vi "STAGE+mono+counter_edit22.vi"() -> ()   [LabVIEW 2017]
panel:
  out "Timeout":bool
  out "PROGRESS":u8(slide) max=10 step=10 scale=0.0..1.0
  in  "?":enum32{"Scan Data", "Scans", "RT Data"}(tab)
  out "Spectrum":cluster{dbl[], dbl[]}(graph)
  out "Decay":cluster{dbl[], dbl[]}[](graph)
  in  "Collect Data!":bool
  out "Waveform Graph":waveform(dbl)[](graph)
  out "?":i32(knob) scale=0.0..1000000.0
  out "Photon Counts":dbl
  in  "Wavelength":dbl
  in  "Show Real Time Data":bool
  in  "?":enum32{"DELAY", "COUNTER", "MONO", "PLOT"}(tab)
  in  "Data File Path":path
  out "Final time [ps]":dbl
  out "Current time [ps]":dbl
  out "Initial time [ps]":dbl
  in  "Set this as t0":bool
  in  "Axis":i32=1
  in  "Motor ON":bool
  in  "Motor OFF":bool
  out "Current Position [mm]":dbl
  out "Final Position [mm]":dbl
  in  "Data Points":i32=100
  out "Current Point":i32
  in  "Step Size [um]":i32=10
  in  "Target [mm]":dbl format="%.3f"
  in  "Move":bool
  out "Initial position [mm]":dbl
  in  "GPIB address":string="23"
  in  "Count Mode":u16(ring) items=["A,B for Preset T", "A-B for Preset T", "A+B for Preset T", "A for Preset B"]
  in  "Trigger mode":u16(ring) items=["10 MHz"=0, "Input 2"=2, "Input T"=3]
  in  "Channel A Input":u16(ring)=1 items=["10 MHz", "Input 1"]
  in  "Channel B Input":u16(ring)=2 items=["Input 1"=1, "Input 2"=2]
  in  "Number of Measurements\n to take at one point/ Number of Periods":u16=1 min=1 max=2000 step=1
  in  "Time between measurements\n at one point (s)/Dwell Time":dbl=0.002 min=0.002 max=60.0 step=0.001
  in  "gate mode (CW:0)":i16(slide) scale=0.0..2.0 scale format="%.2f"
  out "Counts":i32
  in  "Integrating time \nin 10^-7 sec":dbl=10000000.0
  in  "Discriminator Level (mV)":dbl min=-300.0 max=300.0 step=0.2
  in  "Discriminator Slope":bool
  in  "Channel":i16 min=0 max=2 step=1
  out "Grating #":dbl
  out "Blaze angle":dbl
  out "Grooves/mm":dbl
  out "Mono port":T1(ring)
  out "Time delay":u32=450000 min=1
  in  "Step size":dbl=10.0 min=0.0
  in  "Scan to":i32=4000
  in  "Scan from":i32=2600
  out "Current wavelength":dbl
  in  "?":bool
  in  "Array":dbl[](array[numeric])
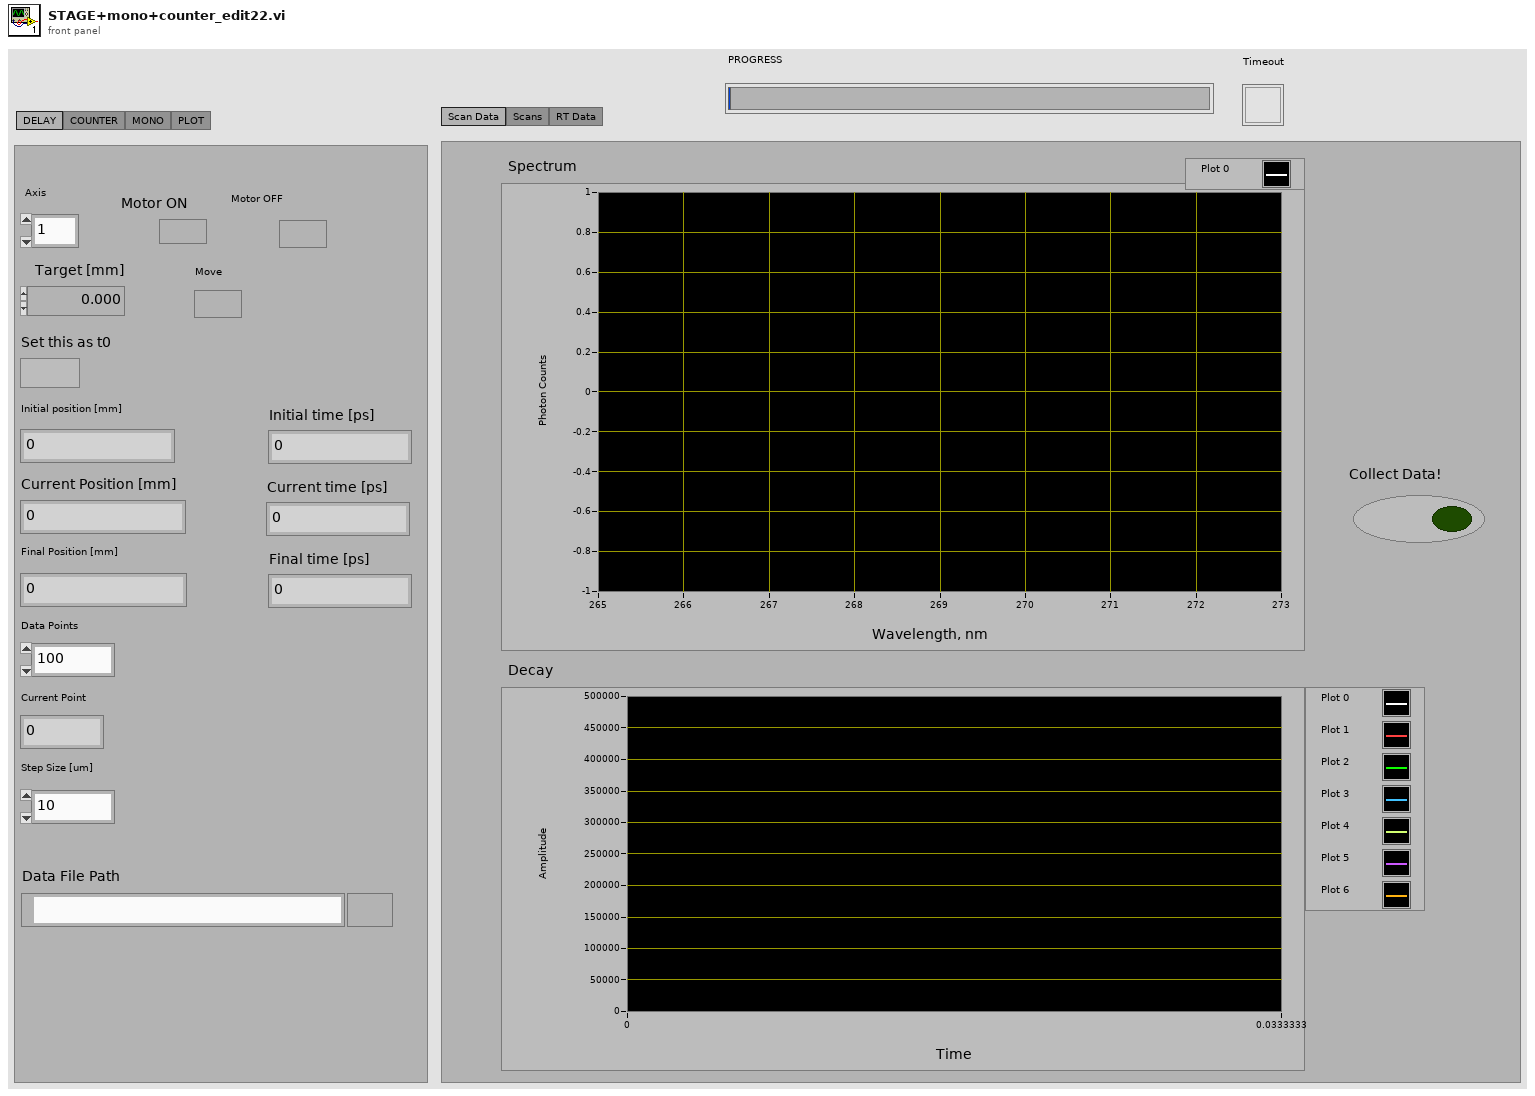
[diagram p1: front panel]
types:
  T1 = enum8{"COM 1", "COM 2", "COM 3", "COM 4", "COM 5", "COM 6", "COM 7", "COM 8", "COM 9"}
  T2 = cluster{"input XON/XOFF":bool, "input HW Handshake":bool, "input alt HW HShk":bool, "output XON/XOFF":bool, "output HW Handshake":bool, "output alt HW HShk":bool, "XOFF byte":u8, "XON byte":u8, "parity error byte":u16}
  T3 = enum16{"no parity", "odd parity", "even parity", "mark parity", "space parity"}
  T4 = enum16{"open", "replace", "create", "open or create", "replace or create", "replace or create with confirmation"}
  T5 = typedef "NI_Matrix.lvlib/RealMatrix.ctl" = dbl[][]
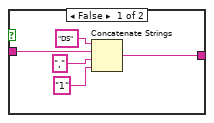
[diagram p3: hidden frame]
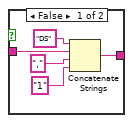
[diagram p5: hidden frame]
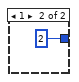
[diagram p9: hidden frame]
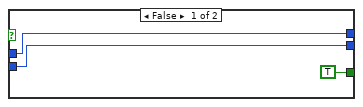
[diagram p10: hidden frame]
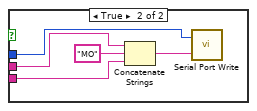
[diagram p11: hidden frame]
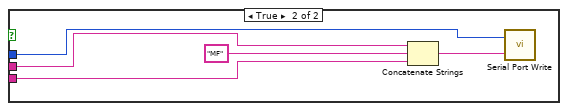
[diagram p12: hidden frame]
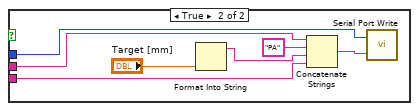
[diagram p13: hidden frame]
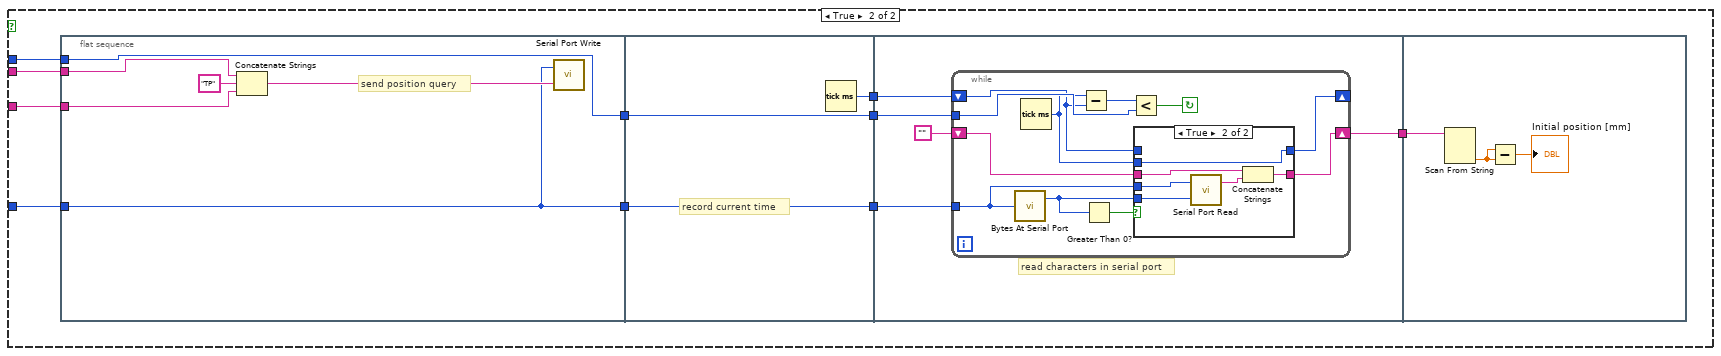
[diagram p14: hidden frame]
diagram:
  (unwired) FALSE
  w28 = u32 19200  # baud rate
  w27 = u16 8  # data bits
  w26 = enum16{"1 bit", "1.5 bits", "2 bits"}."1 bit"  # stop bits
  w30 = T3."no parity"  # parity
  w6 = 4  # 0=COM1 so n=COM(n+1)
  w29 = u16 1024  # buffer size
  n1 = flat-sequence {
    tunnel: [w33] -> w21
    tunnel: [w32] -> w20
    frame #0 {
      n2 = call "CM Com Read ini.vi"() -> ("Mono port"=w32:T1, "time delay1"=w33:u32)  [unwired: 7 in]
    }
  }
  n3 = call "CM Serial Port Setup.vi"("COM port"=w20, "time delay"=w21) -> ("time delay1"=w16:u32, "DK port Out"=w17:T1, "error code"=w19:i32)  [unwired: 7 in]
  n4 = Equal To 0?(x=w19) -> (x = 0?=w18:bool)
  n5 = case shown="True" w18 {
    tunnel: w17 -> [w36 w39]
    tunnel: w16 -> [w35 w38]
    tunnel: [w36 w39] -> w3
    tunnel: [w35 w38] -> w2
    tunnel: [TRUE FALSE] -> w1
    frame False {
    }
    frame True {
      n6 = call "CM Com Write ini.vi"("time delay1"=w39, "Mono port"=w38) -> ()  [unwired: 7 in]
      n7 = local write "Mono port"(w39) -> ()
      n8 = local write "Time delay"(w38) -> ()
    }
  }
  n9 = call <vilib>:"Serial Port Init.vi"("flow control etc."=T2 {"input XON/XOFF"=FALSE, "input HW Handshake"=FALSE, "input alt HW HShk"=FALSE, "output XON/XOFF"=FALSE, "output HW Handshake"=FALSE, "output alt HW HShk"=FALSE, "XOFF byte"=13, "XON byte"=11, "parity error byte"=0}, "parity"=w30, "buffer size"=w29, "stop bits"=w26, "data bits"=w27, "baud rate"=w28, "port number"=w6) -> ("error code"=w25:i32)
  n10 = Concatenate Strings("\r", "\n") -> (w22:string)
  n11 = while {
    tunnel: w2 -> [w42]
    tunnel: w3 -> [w41]
    stop <- TRUE continue-if-true
    n12 = case shown="True" "?" {
      tunnel: w42 -> [_ w45]
      tunnel: w41 -> [_ w44]
      frame False {
      }
      frame True {
        n13 = Two Button Dialog(message="Do you want to change grating?", 1:"No" ("F button name (\"Cancel\")"), 2:"Yes" ("T button name (\"OK\")")) -> (T button?=w46:bool)
        n14 = case shown="True" w46 {
          tunnel: w45 -> [_ w51]
          tunnel: w44 -> [_ w50]
          frame False {
          }
          frame True {
            n15 = Two Button Dialog(message="Disable voltage from PMT", 1:"Do not swich grating" ("F button name (\"Cancel\")"), 2:"Done" ("T button name (\"OK\")")) -> (T button?=w52:bool)
            n16 = case shown="True" w52 {
              tunnel: w51 -> [_ w64]
              tunnel: w50 -> [_ w63]
              frame False {
              }
              frame True {
                n17 = flat-sequence {
                  tunnel: w64 -> [w68]
                  tunnel: [w68] -> w58
                  tunnel: w63 -> [w67]
                  tunnel: [w67] -> w57
                  tunnel: [w65] -> w56
                  tunnel: w58 -> [w73]
                  tunnel: [w73] -> w61
                  tunnel: w57 -> [w74]
                  tunnel: [w74] -> w60
                  tunnel: w56 -> [w72]
                  tunnel: [w72] -> w59
                  tunnel: w61 -> [w78]
                  tunnel: w60 -> [w79]
                  tunnel: [w77] -> w62
                  tunnel: w59 -> [w77]
                  frame #0 {
                    n18 = local read "Grating #"() -> (w66:dbl)
                    n19 = case shown="2, Default" w66 {
                      tunnel: [1 2] -> w65
                      frame 2, Default {
                      }
                      frame 1 {
                      }
                    }
                    n20 = call "Select11x2.vi"("time delay"=w68, "NEW GRT?"=w65, "port number"=w67) -> ()  [unwired: 3 out]
                  }
                  frame #1 {
                    n21 = call "Query11x.vi"("port number"=w74, "QUERY"=u16 2, "time delay"=w73) -> ("STATUS MESSAGE"=w71:u16)  [unwired: 3 out]
                    n22 = local write "Grooves/mm"(w71) -> ()
                  }
                  frame #2 {
                    n23 = Divide(x=w78, y=i16 100 ("device (1)")) -> (x/y=w80:dbl)
                    n24 = call "Query11x.vi"("port number"=w79, "QUERY"=u16 3, "time delay"=w80) -> ("STATUS MESSAGE"=w76:u16)  [unwired: 3 out]
                    n25 = local write "Blaze angle"(w76) -> ()
                  }
                }
                n26 = local write "Grating #"(w62) -> ()
              }
            }
          }
        }
      }
    }
  }
  n27 = while {
    tunnel: w6 -> [w97]
    tunnel: w22 -> [w98]
    tunnel: w25 -> [_]
    tunnel: "Axis" -> [w95]
    stop <- TRUE continue-if-true
    w96 = u32 200  # timeout
    n28 = Format Into String(w95) -> (resulting string=w99:string)  [unwired: 3 in, 1 out]
    n29 = flat-sequence {
      tunnel: w99 -> [w104]
      tunnel: w98 -> [w103]
      tunnel: w97 -> [w105]
      tunnel: w96 -> [w102]
      tunnel: [w104] -> w94
      tunnel: [w103] -> w93
      tunnel: [w105] -> w92
      tunnel: [w102] -> w91
      tunnel: w94 -> [w115]
      tunnel: w93 -> [w114]
      tunnel: w92 -> [w116]
      tunnel: w91 -> [w112]
      tunnel: [w115] -> w90
      tunnel: [w114] -> w89
      tunnel: [w116] -> w88
      tunnel: [w112] -> w87
      tunnel: w90 -> [w125]
      tunnel: w89 -> [w124]
      tunnel: w88 -> [w126]
      tunnel: w87 -> [w122]
      tunnel: [w125] -> w86
      tunnel: [w124] -> w85
      tunnel: [w126] -> w84
      tunnel: [w122] -> w83
      tunnel: w86 -> [w138]
      tunnel: w85 -> [w135]
      tunnel: w84 -> [w137]
      tunnel: w83 -> [w136]
      frame #0 {
        n30 = case shown="False" "Motor ON" {
          tunnel: w105 -> [_ w111]
          tunnel: w104 -> [_ w108]
          tunnel: w103 -> [_ w107]
          frame False {
          }
          frame True {
            n31 = Concatenate Strings(w108, "MO" ("Substring"), w107) -> (w109:string)
            n32 = call <vilib>:"Serial Port Write.vi"("string to write"=w109, "port number"=w111) -> ()  [unwired: 1 out]
          }
        }
      }
      frame #1 {
        n33 = case shown="False" "Motor OFF" {
          tunnel: w116 -> [_ w121]
          tunnel: w115 -> [_ w118]
          tunnel: w114 -> [_ w117]
          frame False {
          }
          frame True {
            n34 = Concatenate Strings(w118, "MF" ("Substring"), w117) -> (w119:string)
            n35 = call <vilib>:"Serial Port Write.vi"("string to write"=w119, "port number"=w121) -> ()  [unwired: 1 out]
          }
        }
      }
      frame #2 {
        n36 = case shown="False" "Move" {
          tunnel: w126 -> [_ w133]
          tunnel: w125 -> [_ w130]
          tunnel: w124 -> [_ w129]
          frame False {
          }
          frame True {
            n37 = Format Into String("Target [mm]") -> (resulting string=w127:string)  [unwired: 3 in, 1 out]
            n38 = Concatenate Strings(w130, "PA" ("Substring"), w127, w129) -> (w131:string)
            n39 = call <vilib>:"Serial Port Write.vi"("string to write"=w131, "port number"=w133) -> ()  [unwired: 1 out]
          }
        }
      }
      frame #3 {
        n40 = case shown="False" "Set this as t0" {
          tunnel: w138 -> [_ w148]
          tunnel: w137 -> [_ w147]
          tunnel: w136 -> [_ w146]
          tunnel: w135 -> [_ w145]
          frame False {
          }
          frame True {
            n41 = flat-sequence {
              tunnel: w148 -> [w152]
              tunnel: w147 -> [w151]
              tunnel: [w151] -> w144
              tunnel: w146 -> [w149]
              tunnel: [w149] -> w143
              tunnel: w145 -> [w150]
              tunnel: w144 -> [w156]
              tunnel: [w156] -> w142
              tunnel: w143 -> [w155]
              tunnel: [w155] -> w141
              tunnel: [w157] -> w140
              tunnel: w142 -> [w162]
              tunnel: w141 -> [w160]
              tunnel: w140 -> [w159]
              tunnel: [w158] -> w139
              tunnel: w139 -> [w184]
              frame #0 {
                # "send position query"
                n42 = Concatenate Strings(w152, "TP" ("Substring"), w150) -> (w153:string)
                n43 = call <vilib>:"Serial Port Write.vi"("string to write"=w153, "port number"=w151) -> ()  [unwired: 1 out]
              }
              frame #1 {
                # "record current time"
                n44 = Tick Count (ms)() -> (millisecond timer value=w157:u32)
              }
              frame #2 {
                # "read characters in serial port"
                n45 = while {
                  shift-left: w159 -> [w163]
                  shift-right: [w164] -> _
                  tunnel: w160 -> [w167]
                  shift-left: "" -> [w170]
                  shift-right: [w169] -> w158
                  tunnel: w162 -> [w171]
                  stop <- w166 continue-if-true
                  n46 = call <vilib>:"Bytes At Serial Port.vi"("port number"=w171) -> ("byte count"=w172:u32)  [unwired: 1 out]
                  n47 = Tick Count (ms)() -> (millisecond timer value=w165:u32)
                  n48 = Subtract(x=w165, y=w163) -> (x-y=w168:u32)
                  n49 = Greater Than 0?(x=w172) -> (x > 0?=w173:bool)
                  n50 = Less?(x=w168, y=w167) -> (x < y?=w166:bool)
                  n51 = case shown="True" w173 {
                    tunnel: w172 -> [_ w181]
                    tunnel: w171 -> [_ w180]
                    tunnel: w170 -> [w175 w178]
                    tunnel: [w175 w177] -> w169
                    tunnel: [w174 w176] -> w164
                    tunnel: w165 -> [_ w176]
                    tunnel: w163 -> [w174 _]
                    frame False {
                    }
                    frame True {
                      n52 = call <vilib>:"Serial Port Read.vi"("requested byte count"=w181, "port number"=w180) -> ("string read"=w179:string)  [unwired: 1 out]
                      n53 = Concatenate Strings(w178, w179) -> (w177:string)
                    }
                  }
                }
              }
              frame #3 {
                n54 = Scan From String(input string=w184) -> (output 1=w182:dbl)  [unwired: 4 in, 3 out]
                n55 = Subtract(x=w182, y=w182) -> (x-y=→"Initial position [mm]":dbl)
              }
            }
          }
        }
      }
    }
    n56 = Wait Until Next ms Multiple(millisecond multiple=u32 50) -> ()  [unwired: 1 out]
  }
  n57 = while {
    tunnel: "GPIB address" -> [w188]
    tunnel: w3 -> [w187]
    tunnel: w2 -> [w186]
    tunnel: w1 -> [w185]
    stop <- TRUE continue-if-true
    n58 = case shown="True" "Show Real Time Data" {
      tunnel: w188 -> [_ w195]
      tunnel: w187 -> [_ w194]
      tunnel: w186 -> [_ w193]
      tunnel: w185 -> [_ w192]
      frame False {
      }
      frame True {
        n59 = flat-sequence {
          tunnel: w195 -> [w224]
          tunnel: "Wavelength" -> [w225]
          tunnel: [w225] -> w206
          tunnel: [w214] -> w205
          tunnel: [w213] -> w204
          tunnel: [w224] -> w203
          tunnel: w193 -> [w217]
          tunnel: w194 -> [w216]
          tunnel: w192 -> [w215]
          tunnel: [w264] -> w202
          tunnel: [w263] -> w201
          tunnel: [w261] -> w200
          tunnel: w206 -> [w259]
          tunnel: w205 -> [w264]
          tunnel: w204 -> [w263]
          tunnel: w203 -> [w261]
          tunnel: w202 -> [w271]
          tunnel: w201 -> [w270]
          tunnel: w200 -> [w265]
          tunnel: [w265] -> w199
          tunnel: w199 -> [w276]
          tunnel: [w276] -> w198
          tunnel: w198 -> [w326]
          tunnel: [w326] -> w197
          tunnel: w197 -> [w327]
          tunnel: [w327] -> w196
          tunnel: w196 -> [w337]
          frame #0 {
            n60 = flat-sequence {
              tunnel: w217 -> [w231]
              tunnel: [w231] -> w223
              tunnel: w216 -> [w233]
              tunnel: [w233] -> w222
              tunnel: w215 -> [w229]
              tunnel: [w229] -> w221
              tunnel: w223 -> [w237]
              tunnel: [w237] -> w212
              tunnel: w222 -> [w238]
              tunnel: [w238] -> w210
              tunnel: w221 -> [w235]
              tunnel: [w235] -> w208
              tunnel: w212 -> [w242]
              tunnel: [w242] -> w211
              tunnel: w210 -> [w241]
              tunnel: [w241] -> w209
              tunnel: w208 -> [w240]
              tunnel: [w240] -> w207
              tunnel: w211 -> [w249]
              tunnel: [w249] -> w220
              tunnel: w209 -> [w246]
              tunnel: [w246] -> w219
              tunnel: w207 -> [w244]
              tunnel: [w244] -> w218
              tunnel: w220 -> [w252]
              tunnel: w219 -> [w253]
              tunnel: w218 -> [_]
              tunnel: [w253] -> w214
              tunnel: [w252] -> w213
              frame #0 {
                n61 = call "Query11x.vi"("port number"=w233, "QUERY"=u16 0, "time delay"=w231) -> ("timeout"=w230:bool, "STATUS MESSAGE"=w228:u16)  [unwired: 2 out]
                n62 = local write "Timeout"(w230) -> ()
                n63 = Divide(x=w228, y=10 ("Numeric")) -> (x/y=w226:dbl)
                n64 = local write "Current wavelength"(w226) -> ()
              }
              frame #1 {
                n65 = call "Query11x.vi"("port number"=w238, "QUERY"=u16 2, "time delay"=w237) -> ("timeout"=w236:bool, "STATUS MESSAGE"=w234:u16)  [unwired: 2 out]
                n66 = local write "Timeout"(w236) -> ()
                n67 = local write "Grooves/mm"(w234) -> ()
              }
              frame #2 {
              }
              frame #3 {
                n68 = Divide(x=w249, y=i16 100 ("device (1)")) -> (x/y=w247:dbl)
                n69 = call "Query11x.vi"("port number"=w246, "QUERY"=u16 3, "time delay"=w247) -> ("timeout"=w245:bool, "STATUS MESSAGE"=w243:u16)  [unwired: 2 out]
                n70 = local write "Timeout"(w245) -> ()
                n71 = local write "Blaze angle"(w243) -> ()
              }
              frame #4 {
                n72 = Divide(x=w252, y=i16 100 ("device (1)")) -> (x/y=w255:dbl)
                n73 = call "Query11x.vi"("port number"=w253, "QUERY"=u16 4, "time delay"=w255) -> ("timeout"=w254:bool, "STATUS MESSAGE"=w251:u16)  [unwired: 2 out]
                n74 = local write "Timeout"(w254) -> ()
                n75 = local write "Grating #"(w251) -> ()
              }
            }
          }
          frame #1 {
            n76 = Multiply(x=w259, y=1) -> (x*y=w258:dbl)
            n77 = call "Goto11x.vi"("time delay"=w263, "WAVELENGTH"=w258, "port number"=w264) -> ("timeout"=w262:bool)  [unwired: 2 out]
            n78 = local write "Timeout"(w262) -> ()
          }
          frame #2 {
            # "set counter time in 10^-7 seconds in CW"
            n79 = call "Query11x.vi"("port number"=w271, "QUERY"=0, "time delay"=w270) -> ("timeout"=w269:bool, "STATUS MESSAGE"=w268:u16)  [unwired: 2 out]
            n80 = local write "Timeout"(w269) -> ()
            n81 = Divide(x=w268, y=1) -> (x/y=w267:dbl)
            n82 = local write "Current wavelength"(w267) -> ()
          }
          frame #3 {
            # "Configures discriminator."
            n83 = flat-sequence {
              tunnel: w276 -> [w283]
              tunnel: [w283] -> w282
              tunnel: [w290] -> w281
              tunnel: [w288] -> w280
              tunnel: w275 -> [w289]
              tunnel: w282 -> [w288]
              tunnel: w277 -> [w287]
              tunnel: w281 -> [w309]
              tunnel: [w310] -> w279
              tunnel: w280 -> [w308]
              tunnel: [w308] -> w278
              tunnel: w277 -> [w306]
              tunnel: w279 -> [w322]
              tunnel: w278 -> [w321]
              tunnel: w273 -> [w316]
              tunnel: w277 -> [w315]
              frame #0 {
                # "Flush I/O buffers."
                n84 = for {
                  N: 5 -> [_]
                  tunnel: w283 -> [w285]
                  n85 = GPIB Write(0:w285, 1:"\r") -> ()  [unwired: 3 in, 2 out]
                }
              }
              frame #1 {
                # "Set discriminator slope."
                n86 = case shown="True" w289 {
                  tunnel: [w296 w301] -> w291
                  tunnel: w287 -> [w295 w300]
                  frame False {
                    n87 = Concatenate Strings("DS", w295, ",", "1") -> (w296:string)
                  }
                  frame True {
                    n88 = Concatenate Strings("DS", w300, ",", "0") -> (w301:string)
                  }
                }
                n89 = GPIB Write(0:w288, 1:w291, 2:5) -> (6:w290:errorcluster)  [unwired: 2 in, 1 out]
              }
              frame #2 {
                # "Set discriminator mode to fixed."
                n90 = Concatenate Strings("DM", w306, ",", "0") -> (w305:string)
                n91 = GPIB Write(0:w308, 1:w305, 2:5, 3:w309) -> (6:w310:errorcluster)  [unwired: 1 in, 1 out]
              }
              frame #3 {
                # "Set discriminator level.\nMust be between +300 and -300 mV."
                n92 = Divide(x=w316, y=1000.0) -> (x/y=w324:dbl)
                n93 = Number To Fractional String(number=w324, precision (6)=i16 4) -> (F-format string=w313:string)  [unwired: 2 in]
                n94 = Concatenate Strings("DL", w315, ",", w313) -> (w320:string)
                n95 = GPIB Write(0:w321, 1:w320, 2:5, 3:w322) -> (6:w317:errorcluster)  [unwired: 1 in, 1 out]
                n96 = call <vilib>:"General Error Handler.vi"("type of dialog (OK msg:1)"=1, "error in (no error)"=w317) -> ()  [unwired: 9 in, 5 out]
              }
            }
            n97 = local read "Discriminator Slope"() -> (w275:bool)
            n98 = local read "Channel"() -> (w274:i16)
            n99 = Number To Decimal String(number=w274) -> (decimal integer string=w277:string)  [unwired: 1 in]
            n100 = local read "Discriminator Level (mV)"() -> (w273:dbl)
          }
          frame #4 {
            n101 = call "Start.vi"("GPIB Address"=w326) -> ()  [unwired: 9 in]
          }
          frame #5 {
            # "Wait for Scan to Finish"
            n102 = for {
              N: 1 -> [_]
              tunnel: w327 -> [w329]
              n103 = while {
                tunnel: w329 -> [w330]
                stop <- w332 stop-if-true
                n104 = call "ScanDone.vi"("Wait (ms)"=1000, "GPIB Address"=w330) -> ("Scan Finished?"=w332:bool)
              }
            }
          }
          frame #6 {
            n105 = call "Read Data.vi"("Channel Number"=0, "GPIB Address"=w337, "Number of Datapoints"=1) -> ("Data"=w338:i32[])
            n106 = property class="Knob (strict)"("Scale.Increment"=1000, "Scale.Maximum"=1000000, "Scale.Minimum"=0) -> ()  [unwired: 2 in, 2 out]
            n107 = Index Array(array=w338, index=0) -> (element=→"Photon Counts" →"?":i32)
          }
        }
      }
    }
  }
  n108 = while {
    tunnel: "Axis" -> [w350]
    tunnel: w6 -> [w349]
    tunnel: "GPIB address" -> [w348]
    tunnel: "Integrating time \nin 10^-7 sec" -> [w347]
    tunnel: w2 -> [w346]
    tunnel: w3 -> [w345]
    tunnel: w1 -> [w344]
    stop <- TRUE continue-if-true
    n109 = case shown="True" "Collect Data!" {
      selector: "Collect Data!" -> [_ w351]
      tunnel: w350 -> [_ w359]
      tunnel: w349 -> [_ w358]
      tunnel: w348 -> [_ w357]
      tunnel: w348 -> [_ w355]
      tunnel: w347 -> [_ w354]
      tunnel: w346 -> [_ w353]
      tunnel: w345 -> [_ w356]
      tunnel: w344 -> [_ w352]
      frame False {
      }
      frame True {
        n110 = flat-sequence {
          tunnel: w359 -> [w379]
          tunnel: w358 -> [w377]
          tunnel: w357 -> [w376]
          tunnel: w356 -> [w375]
          tunnel: w355 -> [w374]
          tunnel: w354 -> [w371]
          tunnel: w353 -> [w364]
          tunnel: w352 -> [w363]
          tunnel: w351 -> [_]
          frame #0 {
            w384 = 1000000000000.0
            w389 = 1000
            w390 = 300000000
            w396 = 1
            n111 = Multiply(x="Step Size [um]", y="Data Points") -> (x*y=w393:i32)
            n112 = Divide(x="Step Size [um]", y=1000.0) -> (x/y=w402:dbl)
            n113 = local read "Initial position [mm]"() -> (w381:dbl)
            n114 = Increment(x="Data Points") -> (x+1=w411:i32)
            n115 = Multiply(x="Scan to", y=w396) -> (x*y=w370:i32)
            n116 = Multiply(x="Scan from", y=w396) -> (x*y=w369:i32)
            n117 = Divide(x=w393, y=1000) -> (x/y=w392:dbl)
            n118 = To Time Stamp(1:w369) -> (0:w399:timestamp)
            n119 = Multiply(x=w370, y=1) -> (x*y=w408:i32)
            n120 = Multiply(x=1, y=w369) -> (x*y=w373:i32)
            n121 = Divide(x=w402, y=1000.0) -> (x/y=w403:dbl)
            n122 = for {
              N: w411 -> [_]
              tunnel: w402 -> [w809]
              tunnel: w381 -> [w807]
              tunnel: [w800] -> w410 mode=indexing
              i -> [w808]
              # "distances"
              n123 = Multiply(x=w809, y=w808) -> (x*y=w806:dbl)
              n124 = Add(x=w807, y=w806) -> (x+y=w805:dbl)
              n125 = Divide(x=w805, y=1000) -> (x/y=w799:dbl)
              n126 = Divide(x=w799, y=300000000) -> (x/y=w802:dbl)
              n127 = Multiply(x=w802, y=1000000000000.0) -> (x*y=w800:dbl)
            }
            n128 = Subtract(x=w408, y=w373) -> (x-y=w414:i32)
            n129 = Divide(x=w381, y=w389) -> (x/y=w387:dbl)
            n130 = Add(x=w381, y=w392) -> (x+y=w383:dbl)
            "Final Position [mm]" <- w383
            n131 = property on="Waveform Graph" class="WFGraph (strict)"("XScale.Increment"="Step size", "XScale.Maximum"=w370, "XScale.Minimum"=w369) -> ()  [unwired: 2 in, 2 out]
            n132 = Divide(x=w383, y=w389) -> (x/y=w388:dbl)
            n133 = Divide(x=w414, y="Step size") -> (x/y=w413:dbl)
            n134 = Divide(x=w387, y=w390) -> (x/y=w386:dbl)
            n135 = Divide(x=w403, y=300000000) -> (x/y=w405:dbl)
            n136 = Bundle By Name("Y"=dbl[] [], "t0"=w399, "dt"="Step size") -> (w398:waveform(dbl))  [unwired: 1 in]
            n137 = Divide(x=w388, y=w390) -> (x/y=w385:dbl)
            n138 = Multiply(x=w405, y=1000000000000.0) -> (x*y=w367:dbl)
            n139 = Multiply(x=w386, y=w384) -> (x*y=w366:dbl)
            "Initial time [ps]" <- w366
            n140 = Build Array(w398) -> (w362:waveform(dbl)[])
            n141 = Round Toward -Infinity(1:w413) -> (0:w372:dbl)
            n142 = Concatenate Strings("\r", "\n") -> (w378:string)
            n143 = Increment(x=w372) -> (x+1=w401:dbl)
            n144 = Multiply(x=w385, y=w384) -> (x*y=w397:dbl)
            "Final time [ps]" <- w397
            n145 = for {
              N: w401 -> [_]
              tunnel: "Step size" -> [w814]
              tunnel: w373 -> [w812]
              tunnel: [w810] -> _ mode=indexing
              i -> [w813]
              # "wavelengths"
              n146 = Multiply(x=w814, y=w813) -> (x*y=w811:dbl)
              n147 = Add(x=w812, y=w811) -> (x+y=w810:dbl)
            }
            n148 = for {
              N: "Data Points" -> [w438]
              tunnel: w381 -> [w479]
              tunnel: "Step Size [um]" -> [w475]
              tunnel: w379 -> [w472]
              tunnel: w378 -> [w469]
              tunnel: w377 -> [w470]
              tunnel: w376 -> [w468]
              tunnel: w375 -> [w466]
              tunnel: w374 -> [w467]
              tunnel: w373 -> [w429]
              tunnel: "Step size" -> [w461]
              tunnel: w372 -> [w460]
              tunnel: w371 -> [w459]
              tunnel: w370 -> [w424]
              tunnel: w369 -> [w423]
              tunnel: "Step size" -> [w425]
              tunnel: w367 -> [w440]
              tunnel: w366 -> [w457]
              shift-right: [w439] -> _
              shift-left: dbl[] [] -> [w435]
              tunnel: w364 -> [w452]
              tunnel: w375 -> [w451]
              tunnel: w363 -> [w450]
              shift-right: [w445] -> _
              shift-left: w362 -> [w446]
              shift-right: [w433] -> _
              shift-left: dbl[][] [] -> [w432]
              shift-right: [w421] -> _
              shift-left: dbl[][] [] -> [w419]
              i -> [w427]
              w449 = dbl[] []
              n149 = property on="PROGRESS" class="Slide (strict)"("Scale.Increment"=1, "Scale.Maximum"=w438, "Scale.Minimum"=0) -> ()  [unwired: 2 in, 2 out]
              n150 = stacked-sequence {
                tunnel: w466 -> [w782]
                tunnel: w467 -> [_]
                frame #0 {
                  n151 = call <vilib>:"Close Serial Driver.vi"("port number"=w782) -> ()  [unwired: 1 out]
                  n152 = GPIB Misc(0:"loc 23" ("command string")) -> ()  [unwired: 1 in, 3 out]
                }
              }
              n153 = property on="Waveform Graph" class="WFGraph (strict)"("XScale.Increment"=w425, "XScale.Maximum"=w424, "XScale.Minimum"=w423) -> ()  [unwired: 2 in, 2 out]
              n154 = Multiply(x=w440, y=w427) -> (x*y=w458:dbl)
              n155 = Number To Decimal String(number=w459) -> (decimal integer string=w464:string)  [unwired: 1 in]
              n156 = Add(x=1, y=w427) -> (x+y=→"PROGRESS":i32)
              n157 = Divide(x=w475, y=1000) -> (x/y=w474:dbl)
              n158 = Add(x=w457, y=w458) -> (x+y=w436:dbl)
              n159 = Concatenate Strings("CP 2,", w464) -> (w462:string)
              n160 = Multiply(x=w474, y=w427) -> (x*y=w478:dbl)
              n161 = Build Array (concatenate)(w435, w436) -> (w437:dbl[])
              n162 = Add(x=w479, y=w478) -> (x+y=w477:dbl)
              n163 = Format Into String(w472) -> (resulting string=w471:string)  [unwired: 3 in, 1 out]
              n164 = GPIB Write(0:w468, 1:w462, 2:i16 5 ("mode (0)")) -> ()  [unwired: 2 in, 2 out]
              n165 = flat-sequence {
                tunnel: w477 -> [w785]
                tunnel: [w785] -> w473
                tunnel: w469 -> [w787]
                tunnel: w471 -> [w786]
                tunnel: w470 -> [w783]
                tunnel: w473 -> [w796]
                tunnel: [w791] -> w422
                frame #0 {
                  n166 = Format Into String(w785) -> (resulting string=w784:string)  [unwired: 3 in, 1 out]
                  n167 = Wait (ms)(milliseconds to wait=u32 100) -> ()  [unwired: 1 out]
                  n168 = Concatenate Strings(w786, "PA" ("Substring"), w784, w787) -> (w789:string)
                  n169 = call <vilib>:"Serial Port Write.vi"("string to write"=w789, "port number"=w783) -> ()  [unwired: 1 out]
                }
                frame #1 {
                  n170 = Divide(x=w796, y=1000) -> (x/y=w794:dbl)
                  n171 = Wait (ms)(milliseconds to wait=u32 1000) -> ()  [unwired: 1 out]
                  n172 = Divide(x=w794, y=300000000) -> (x/y=w793:dbl)
                  n173 = Multiply(x=w793, y=1000000000000.0) -> (x*y=w791:dbl)
                  "Current time [ps]" <- w791
                  "Current Position [mm]" <- w796
                }
              }
              n174 = Add(x=w427, y=1) -> (x+y=w426:i32)
              n175 = flat-sequence {
                tunnel: w468 -> [w505]
                tunnel: w429 -> [w504]
                tunnel: w461 -> [w503]
                tunnel: w460 -> [w502]
                tunnel: w424 -> [w501]
                tunnel: w423 -> [w500]
                tunnel: w449 -> [w499]
                tunnel: w449 -> [w498]
                tunnel: w425 -> [w497]
                tunnel: w452 -> [w496]
                tunnel: w451 -> [w495]
                tunnel: w450 -> [w494]
                tunnel: [w492] -> w448
                tunnel: [w493] -> _
                tunnel: [w492] -> w447
                tunnel: w426 -> [w491]
                tunnel: w422 -> [w490]
                tunnel: [w489] -> w420
                tunnel: w419 -> [w488]
                tunnel: w448 -> [w760]
                tunnel: [w763] -> w434
                tunnel: [w762] -> w431
                tunnel: [w761] -> w421
                tunnel: w420 -> [w761]
                frame #0 {
                  # "step size"
                  n176 = while {
                    tunnel: w505 -> [w545]
                    tunnel: w504 -> [w568]
                    tunnel: w503 -> [w538]
                    tunnel: w502 -> [w567]
                    tunnel: w501 -> [w541]
                    tunnel: w500 -> [w540]
                    tunnel: w497 -> [w542]
                    shift-right: [w564] -> w492
                    shift-left: w498 -> [w563]
                    shift-right: [w559] -> w493
                    shift-left: w499 -> [w566]
                    tunnel: w496 -> [w549]
                    tunnel: w495 -> [w548]
                    tunnel: w494 -> [w547]
                    tunnel: w491 -> [w526]
                    tunnel: w490 -> [w514]
                    shift-right: [w507] -> w489
                    shift-left: w488 -> [w506]
                    i -> [w534]
                    stop <- w536 stop-if-true
                    n177 = property on="Spectrum" class="XYGraph (strict)"("XScale.Increment"=w542, "XScale.Maximum"=w541, "XScale.Minimum"=w540) -> ()  [unwired: 2 in, 2 out]
                    n178 = Multiply(x=1, y=w538) -> (x*y=w537:dbl)
                    n179 = Greater Or Equal?(x=w534, y=w567) -> (x >= y?=w536:bool)
                    n180 = Multiply(x=w534, y=w537) -> (x*y=w569:dbl)
                    n181 = Add(x=w569, y=w568) -> (x+y=w546:dbl)
                    n182 = Add(x=w534, y=1) -> (x+y=w527:i32)
                    n183 = Build Array (concatenate)(w566, w546) -> (w565:dbl[])
                    n184 = flat-sequence {
                      tunnel: w545 -> [w590]
                      tunnel: w546 -> [w591]
                      tunnel: [w591] -> w553
                      tunnel: [w580] -> w552
                      tunnel: [w579] -> w551
                      tunnel: [w590] -> w550
                      tunnel: w549 -> [w583]
                      tunnel: w548 -> [w582]
                      tunnel: w547 -> [w581]
                      tunnel: [w572] -> w528
                      tunnel: w527 -> [w572]
                      tunnel: [w571] -> w515
                      tunnel: w514 -> [w571]
                      tunnel: w506 -> [w570]
                      tunnel: [w570] -> w513
                      tunnel: [w633] -> w558
                      tunnel: [w632] -> w557
                      tunnel: [w630] -> w556
                      tunnel: w553 -> [w626]
                      tunnel: w552 -> [w633]
                      tunnel: w551 -> [w632]
                      tunnel: w550 -> [w630]
                      tunnel: [w627] -> w529
                      tunnel: w528 -> [w627]
                      tunnel: [w626] -> w521
                      tunnel: [w625] -> w516
                      tunnel: w515 -> [w625]
                      tunnel: w513 -> [w624]
                      tunnel: [w624] -> w512
                      tunnel: w558 -> [w644]
                      tunnel: w557 -> [w643]
                      tunnel: w556 -> [w638]
                      tunnel: [w638] -> w544
                      tunnel: [w637] -> w530
                      tunnel: w529 -> [w637]
                      tunnel: [w636] -> w522
                      tunnel: w521 -> [w636]
                      tunnel: [w635] -> w517
                      tunnel: w516 -> [w635]
                      tunnel: w512 -> [w634]
                      tunnel: [w634] -> w511
                      tunnel: w544 -> [w650]
                      tunnel: [w650] -> w543
                      tunnel: [w649] -> w531
                      tunnel: w530 -> [w649]
                      tunnel: [w648] -> w523
                      tunnel: w522 -> [w648]
                      tunnel: [w647] -> w518
                      tunnel: w517 -> [w647]
                      tunnel: w511 -> [w646]
                      tunnel: [w646] -> w510
                      tunnel: w543 -> [w707]
                      tunnel: [w707] -> w555
                      tunnel: [w706] -> w532
                      tunnel: w531 -> [w706]
                      tunnel: [w705] -> w524
                      tunnel: w523 -> [w705]
                      tunnel: [w704] -> w519
                      tunnel: w518 -> [w704]
                      tunnel: w510 -> [w703]
                      tunnel: [w703] -> w509
                      tunnel: w555 -> [w712]
                      tunnel: [w712] -> w554
                      tunnel: [w711] -> w533
                      tunnel: w532 -> [w711]
                      tunnel: [w710] -> w525
                      tunnel: w524 -> [w710]
                      tunnel: [w709] -> w520
                      tunnel: w519 -> [w709]
                      tunnel: w509 -> [w708]
                      tunnel: [w708] -> w508
                      tunnel: [w723] -> w561
                      tunnel: w554 -> [w755]
                      tunnel: w533 -> [w721]
                      tunnel: w526 -> [w724]
                      tunnel: w525 -> [w725]
                      tunnel: w520 -> [w727]
                      tunnel: w508 -> [w722]
                      tunnel: [w720] -> w507
                      frame #0 {
                        n185 = flat-sequence {
                          tunnel: w583 -> [w597]
                          tunnel: [w597] -> w589
                          tunnel: w582 -> [w599]
                          tunnel: [w599] -> w588
                          tunnel: w581 -> [w595]
                          tunnel: [w595] -> w587
                          tunnel: w589 -> [w603]
                          tunnel: [w603] -> w578
                          tunnel: w588 -> [w604]
                          tunnel: [w604] -> w576
                          tunnel: w587 -> [w601]
                          tunnel: [w601] -> w574
                          tunnel: w578 -> [w608]
                          tunnel: [w608] -> w577
                          tunnel: w576 -> [w607]
                          tunnel: [w607] -> w575
                          tunnel: w574 -> [w606]
                          tunnel: [w606] -> w573
                          tunnel: w577 -> [w615]
                          tunnel: [w615] -> w586
                          tunnel: w575 -> [w612]
                          tunnel: [w612] -> w585
                          tunnel: w573 -> [w610]
                          tunnel: [w610] -> w584
                          tunnel: w586 -> [w617]
                          tunnel: w585 -> [w618]
                          tunnel: w584 -> [_]
                          tunnel: [w618] -> w580
                          tunnel: [w617] -> w579
                          frame #0 {
                            n186 = call "Query11x.vi"("port number"=w599, "QUERY"=u16 0, "time delay"=w597) -> ("timeout"=w596:bool, "STATUS MESSAGE"=w594:u16)  [unwired: 2 out]
                            n187 = local write "Timeout"(w596) -> ()
                            n188 = Divide(x=w594, y=1 ("Numeric")) -> (x/y=→"Current wavelength":dbl)
                          }
                          frame #1 {
                            n189 = call "Query11x.vi"("port number"=w604, "QUERY"=u16 2, "time delay"=w603) -> ("timeout"=w602:bool, "STATUS MESSAGE"=→"Grooves/mm":u16)  [unwired: 2 out]
                            n190 = local write "Timeout"(w602) -> ()
                          }
                          frame #2 {
                          }
                          frame #3 {
                            n191 = Divide(x=w615, y=i16 100 ("device (1)")) -> (x/y=w613:dbl)
                            n192 = call "Query11x.vi"("port number"=w612, "QUERY"=u16 3, "time delay"=w613) -> ("timeout"=w611:bool, "STATUS MESSAGE"=→"Blaze angle":u16)  [unwired: 2 out]
                            n193 = local write "Timeout"(w611) -> ()
                          }
                          frame #4 {
                            n194 = Divide(x=w617, y=i16 100 ("device (1)")) -> (x/y=w621:dbl)
                            n195 = call "Query11x.vi"("port number"=w618, "QUERY"=u16 4, "time delay"=w621) -> ("timeout"=w620:bool, "STATUS MESSAGE"=→"Grating #":u16)  [unwired: 2 out]
                            n196 = local write "Timeout"(w620) -> ()
                          }
                        }
                      }
                      frame #1 {
                        n197 = Multiply(x=w626, y=1) -> (x*y=w628:dbl)
                        n198 = call "Goto11x.vi"("time delay"=w632, "WAVELENGTH"=w628, "port number"=w633) -> ("timeout"=w631:bool)  [unwired: 2 out]
                        n199 = local write "Timeout"(w631) -> ()
                      }
                      frame #2 {
                        # "set counter time in 10^-7 seconds in CW"
                        n200 = call "Query11x.vi"("port number"=w644, "QUERY"=0, "time delay"=w643) -> ("timeout"=w642:bool, "STATUS MESSAGE"=w641:u16)  [unwired: 2 out]
                        n201 = local write "Timeout"(w642) -> ()
                        n202 = Divide(x=w641, y=1) -> (x/y=w640:dbl)
                        n203 = local write "Current wavelength"(w640) -> ()
                      }
                      frame #3 {
                        # "Configures discriminator."
                        n204 = flat-sequence {
                          tunnel: w650 -> [w660]
                          tunnel: [w660] -> w659
                          tunnel: [w667] -> w658
                          tunnel: [w665] -> w657
                          tunnel: "Discriminator Slope" -> [w666]
                          tunnel: w659 -> [w665]
                          tunnel: w651 -> [w664]
                          tunnel: w658 -> [w686]
                          tunnel: [w687] -> w656
                          tunnel: w657 -> [w685]
                          tunnel: [w685] -> w655
                          tunnel: w651 -> [w683]
                          tunnel: w656 -> [w699]
                          tunnel: w655 -> [w698]
                          tunnel: "Discriminator Level (mV)" -> [w693]
                          tunnel: w651 -> [w692]
                          frame #0 {
                            # "Flush I/O buffers."
                            n205 = for {
                              N: 5 -> [_]
                              tunnel: w660 -> [w662]
                              n206 = GPIB Write(0:w662, 1:"\r") -> ()  [unwired: 3 in, 2 out]
                            }
                          }
                          frame #1 {
                            # "Set discriminator slope."
                            n207 = case shown="True" w666 {
                              tunnel: [w673 w678] -> w668
                              tunnel: w664 -> [w672 w677]
                              frame False {
                                n208 = Concatenate Strings("DS", w672, ",", "1") -> (w673:string)
                              }
                              frame True {
                                n209 = Concatenate Strings("DS", w677, ",", "0") -> (w678:string)
                              }
                            }
                            n210 = GPIB Write(0:w665, 1:w668, 2:5) -> (6:w667:errorcluster)  [unwired: 2 in, 1 out]
                          }
                          frame #2 {
                            # "Set discriminator mode to fixed."
                            n211 = Concatenate Strings("DM", w683, ",", "0") -> (w682:string)
                            n212 = GPIB Write(0:w685, 1:w682, 2:5, 3:w686) -> (6:w687:errorcluster)  [unwired: 1 in, 1 out]
                          }
                          frame #3 {
                            # "Set discriminator level.\nMust be between +300 and -300 mV."
                            n213 = Divide(x=w693, y=1000.0) -> (x/y=w701:dbl)
                            n214 = Number To Fractional String(number=w701, precision (6)=i16 4) -> (F-format string=w690:string)  [unwired: 2 in]
                            n215 = Concatenate Strings("DL", w692, ",", w690) -> (w697:string)
                            n216 = GPIB Write(0:w698, 1:w697, 2:5, 3:w699) -> (6:w694:errorcluster)  [unwired: 1 in, 1 out]
                            n217 = call <vilib>:"General Error Handler.vi"("type of dialog (OK msg:1)"=1, "error in (no error)"=w694) -> ()  [unwired: 9 in, 5 out]
                          }
                        }
                        n218 = Number To Decimal String(number="Channel") -> (decimal integer string=w651:string)  [unwired: 1 in]
                      }
                      frame #4 {
                        n219 = call "Start.vi"("GPIB Address"=w707) -> ()  [unwired: 9 in]
                      }
                      frame #5 {
                        # "Wait for Scan to Finish"
                        n220 = for {
                          N: 1 -> [_]
                          tunnel: w712 -> [w714]
                          n221 = while {
                            tunnel: w714 -> [w715]
                            stop <- w717 stop-if-true
                            n222 = call "ScanDone.vi"("Wait (ms)"=1000, "GPIB Address"=w715) -> ("Scan Finished?"=w717:bool)
                          }
                        }
                      }
                      frame #6 {
                        w726 = 0
                        w734 = "\r\n"
                        n223 = call "Read Data.vi"("Channel Number"=0, "GPIB Address"=w755, "Number of Datapoints"=1) -> ("Data"=w756:i32[])
                        n224 = Index Array(array=w756, index=0) -> (element=w723:i32)
                        "Counts" <- w723
                        n225 = local read "Integrating time \nin 10^-7 sec"() -> (w732:dbl)
                        n226 = Replace Array Subset(array=w722, new element #1=w723, index (row) #1=w721, index (col) #1=w724, new element #2=w725, index (row) #2=w721, index (col) #2=w726, new element #3=w727, index (row) #3=w726, index (col) #3=w724) -> (w720:T5)
                        n227 = Array To Spreadsheet String(delimiter (Tab)=",", array=w720, 3:"%f" ("format string")) -> (spreadsheet string=w733:string)
                        n228 = local read "Blaze angle"() -> (w750:dbl)
                        n229 = local read "Grating #"() -> (w749:dbl)
                        n230 = Multiply(x=w732, y=1e-07) -> (x*y=w731:dbl)
                        n231 = Get Date/Time In Seconds() -> (seconds since 1Jan1904=w744:timestamp)
                        n232 = Format Date/Time String(time format string (%c)="%Y-%b-%d %H:%M:%S", seconds (now)=w744) -> (date/time string=w745:string)  [unwired: 1 in]
                        n233 = Number To Decimal String(number=w731) -> (decimal integer string=w746:string)  [unwired: 1 in]
                        n234 = Number To Decimal String(number=w749) -> (decimal integer string=w747:string)  [unwired: 1 in]
                        n235 = Number To Decimal String(number=w750) -> (decimal integer string=w735:string)  [unwired: 1 in]
                        n236 = call <vilib>:"Space Constant.vi"() -> ("String"=w748:string)
                        n237 = Open/Create/Replace File(file path (use dialog)="Data File Path", operation (0:open)=T4."replace or create") -> (refnum out=w754:refnum<file>)  [unwired: 4 in, 2 out]
                        n238 = Concatenate Strings(w734, "Data was taken on ", w745, w734, "Integration Time is ", w746, w748, "s", w734, "Monochromator gratng # ", w747, "; ", "blazed for ", w735, w748, "nm", w734, w734, w734, w733) -> (w729:string)
                        n239 = Write to Text File(file (use dialog)=w754, text=w729) -> (refnum out=w719:refnum<file>)  [unwired: 2 in, 2 out]
                        n240 = Flush File(refnum=w719) -> (refnum out=w718:refnum<file>)  [unwired: 1 in, 1 out]
                        n241 = Close File(refnum=w718) -> ()  [unwired: 1 in, 2 out]
                      }
                    }
                    n242 = Build Array (concatenate)(w563, w561) -> (w562:dbl[])
                    n243 = Bundle(w565, w562) -> (w560:cluster{dbl[], dbl[]})  [unwired: 1 in]
                    "Spectrum" <- w560
                    n244 = Unbundle(w560) -> (w559:dbl[], w564:dbl[])
                  }
                }
                frame #1 {
                  n245 = Array Size(array="Array") -> (size(s)=w762:i32)
                  n246 = flat-sequence {
                    tunnel: w760 -> [w769]
                    tunnel: "Array" -> [w768]
                    tunnel: w762 -> [w767]
                    tunnel: [w765] -> w763
                    frame #0 {
                      n247 = for {
                        N: w767 -> [_]
                        tunnel: w768 -> [w780]
                        tunnel: w769 -> [w775]
                        shift-right: [w770] -> w765
                        shift-left: dbl[] [] -> [w771]
                        i -> [w773]
                        n248 = local read "Scan from"() -> (w778:i32)
                        n249 = Index Array(array=w780, index=w773) -> (element=w779:dbl)
                        n250 = local read "Step size"() -> (w776:dbl)
                        n251 = Subtract(x=w779, y=w778) -> (x-y=w777:dbl)
                        n252 = Divide(x=w777, y=w776) -> (x/y=w774:dbl)
                        n253 = Index Array(array=w775, index=w774) -> (element=w772:dbl)
                        n254 = Insert Into Array(array=w771, index=w773, new element=w772) -> (w770:dbl[])
                      }
                    }
                  }
                }
              }
              n255 = local read "Scan from"() -> (w443:i32)
              n256 = local read "Step size"() -> (w441:dbl)
              n257 = To Time Stamp(1:w443) -> (0:w442:timestamp)
              n258 = Bundle By Name("Y"=w447, "t0"=w442, "dt"=w441) -> (w444:waveform(dbl))  [unwired: 1 in]
              n259 = Build Array (concatenate)(w446, w444) -> (w445:waveform(dbl)[])
              "Waveform Graph" <- w445
              n260 = for {
                N: w431 -> [_]
                tunnel: [w487] -> w439
                tunnel: w437 -> [w486]
                tunnel: w434 -> [w484]
                tunnel: [w483] -> w433
                tunnel: w432 -> [w485]
                tunnel: [w480] -> w430 mode=indexing
                i -> [w482]
                n261 = Build Array (concatenate)(w485, w484) -> (w483:dbl[][])
                n262 = Index Array(array=w484, index=w482) -> ()  [unwired: 1 out]
                n263 = Index Array(array=w483, index (col)=w482) -> (element=w481:dbl[])  [unwired: 1 in]
                n264 = Bundle(w486, w481) -> (w480:cluster{dbl[], dbl[]})  [unwired: 1 in]
                n265 = Unbundle(w480) -> (w487:dbl[])  [unwired: 1 out]
              }
              "Decay" <- w430
              "Current Point" <- w427
            }
            n266 = property on="Decay" class="XYGraph (strict)"("XScale.Increment"=w367, "XScale.Maximum"=w397, "XScale.Minimum"=w366) -> ()  [unwired: 2 in, 2 out]
            n267 = Build Array (concatenate)(0, w410) -> ()  [unwired: 1 out]
          }
        }
      }
    }
  }
  n268 = call "Configure.vi"("Dwell Time (s)"="Time between measurements\n at one point (s)/Dwell Time", "Channel T Input"="Trigger mode", "Channel B Input"="Channel B Input", "Channel A Input"="Channel A Input", "Integrating time, 10^-7 sec"="Integrating time \nin 10^-7 sec", "gate mode (CW:0)"="gate mode (CW:0)", "Scan End Mode"=FALSE, "Number of Periods"="Number of Measurements\n to take at one point/ Number of Periods", "Count Mode"="Count Mode", "GPIB Address"="GPIB address") -> ()
  "Mono port" <- w20
  "Time delay" <- w21
